vi "pdNormalize_III.vi"(0 "422 Data":T1, 5 "532 Data":T2, 7 "785 Data":T3, 12 "422 PD Cal 3":dbl, 13 "532 PD Cal 3":dbl, 14 "785 PD Cal 3":dbl) -> (4 "pd ts":cluster{dbl, dbl, dbl}(graph), 6 "422 New Array":dbl[](array[numeric]), 8 "532 New Array":dbl[](array[numeric]), 10 "785 New Array":dbl[](array[numeric]))   [LabVIEW 2011]
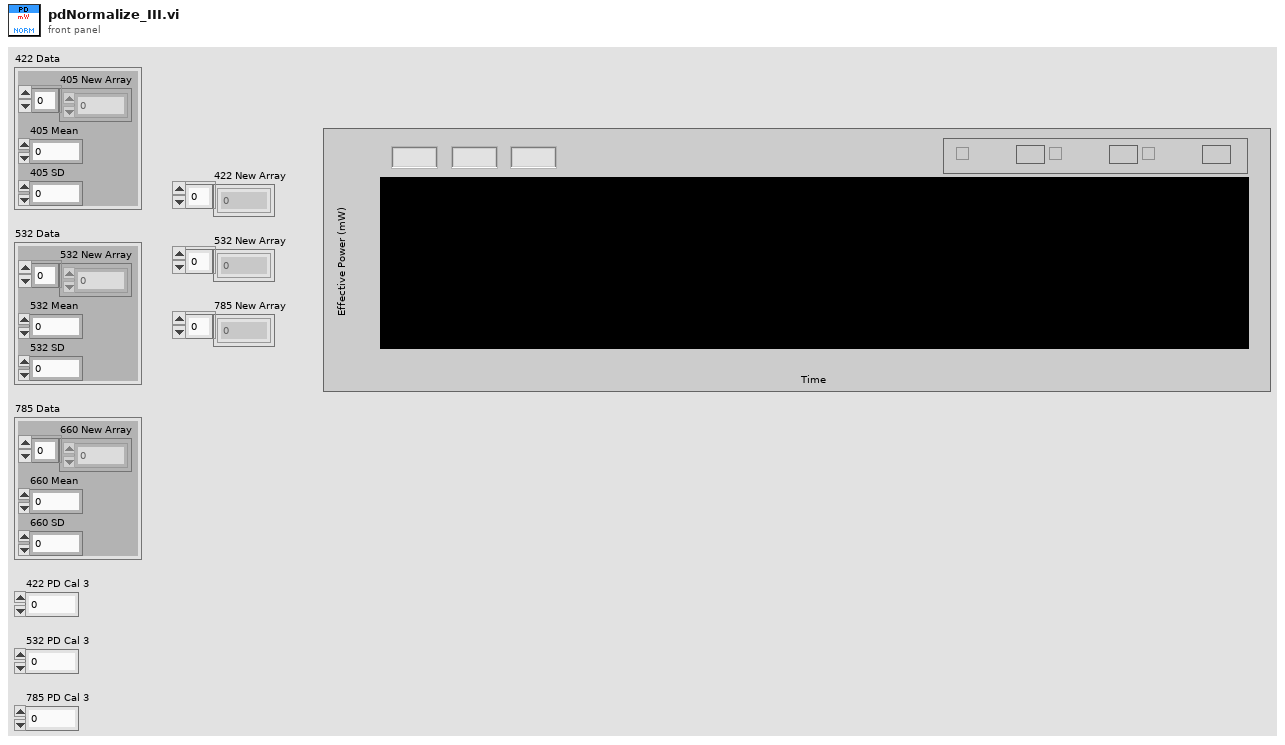
[diagram p1: front panel]
types:
  T1 = cluster{"405 New Array":dbl[], "405 Mean":dbl, "405 SD":dbl}
  T2 = cluster{"532 New Array":dbl[], "532 Mean":dbl, "532 SD":dbl}
  T3 = cluster{"660 New Array":dbl[], "660 Mean":dbl, "660 SD":dbl}
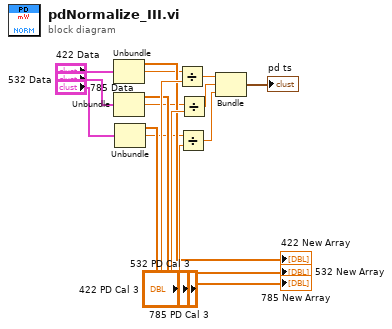
[diagram p0: block diagram]
diagram:
  n1 = Unbundle("422 Data") -> ("405 New Array"=→"422 New Array":dbl[], "405 Mean"=w3:dbl)  [unwired: 1 out]
  n2 = Unbundle("532 Data") -> ("532 New Array"=→"532 New Array":dbl[], "532 Mean"=w5:dbl)  [unwired: 1 out]
  n3 = Unbundle("785 Data") -> ("660 New Array"=→"785 New Array":dbl[], "660 Mean"=w7:dbl)  [unwired: 1 out]
  n4 = Divide(x=w3, y="422 PD Cal 3") -> (x/y=w2:dbl)
  n5 = Divide(x=w7, y="785 PD Cal 3") -> (x/y=w6:dbl)
  n6 = Divide(x=w5, y="532 PD Cal 3") -> (x/y=w4:dbl)
  n7 = Bundle(w2, w4, w6) -> (→"pd ts":cluster{dbl, dbl, dbl})  [unwired: 1 in]
